vi "Remove Connection.vi"(8 "error in (no error)":errorcluster, 10 "Connection Name":string, 11 "VectoService in":refnum<class "VectoInfo.lvclass">) -> (0 "error out":errorcluster, 3 "VectoService out":refnum<class "VectoInfo.lvclass">)   [LabVIEW 2020, in "Vecto.lvlib" / "VectoInfo.lvclass"]
uses:
  VectoInfo.lvclass
  VectoInfo.lvclass/VectoInfo.ctl
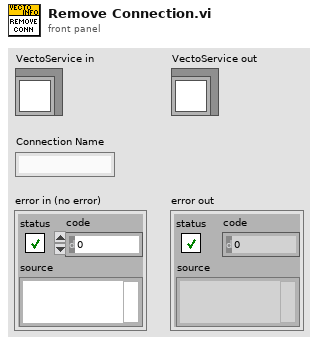
[diagram p1: front panel]
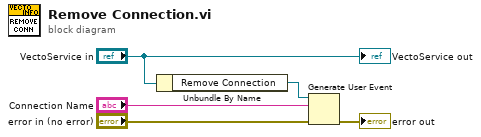
[diagram p0: block diagram]
diagram:
  n1 = Unbundle By Name("VectoService in") -> ("Remove Connection"=w5:refnum<user-event>)
  n2 = Generate User Event(user event=w5, event data cluster="Connection Name", error in="error in (no error)") -> (error out=→"error out":errorcluster)  [unwired: 1 in, 1 out]
  "VectoService out" <- "VectoService in"
